vi "Stage_1_waveform_for_DAQ.vi"(11 "input cluster":T2) -> (2 "DAQ cluster":T1, 3 "Time cluster":cluster{"Total time":dbl, "Time per step":dbl})   [LabVIEW 2016]
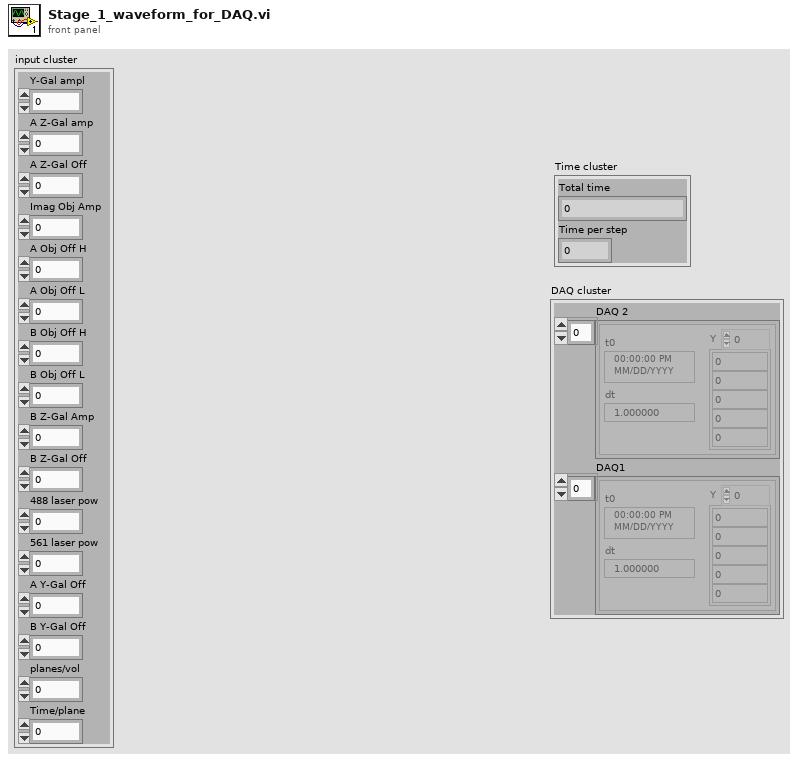
[diagram p1: front panel]
types:
  T1 = cluster{"DAQ1":waveform(dbl)[], "DAQ 2":waveform(dbl)[]}
  T2 = cluster{"Y-Gal ampl":dbl, "A Z-Gal amp":dbl, "A Z-Gal Off":dbl, "Imag Obj Amp":dbl, "A Obj Off H":dbl, "A Obj Off L":dbl, "B Obj Off H":dbl, "B Obj Off L":dbl, "B Z-Gal Amp":dbl, "B Z-Gal Off":dbl, "488 laser pow":dbl, "561 laser pow":dbl, "A Y-Gal Off":dbl, "B Y-Gal Off ":dbl, "planes/vol":dbl, "Time/plane":dbl}
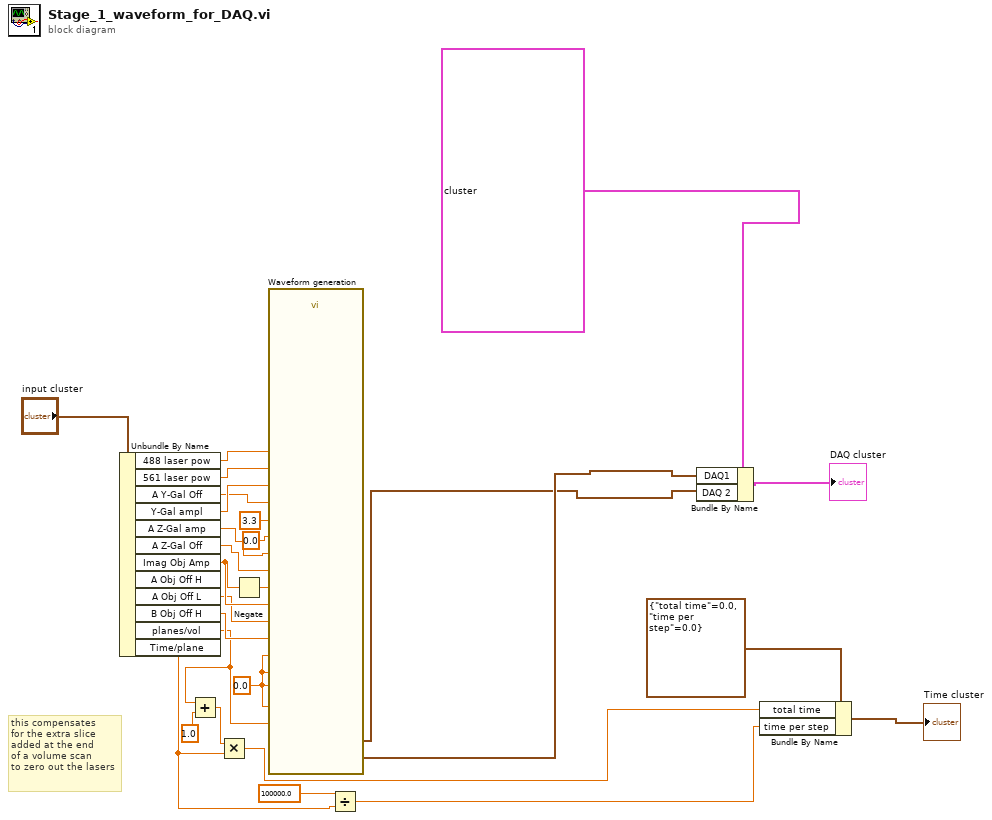
[diagram p0: block diagram]
diagram:
  w27 = 0.0 ("ARM2 Z-offset")
  # "this compensates\nfor the extra slice\nadded at the end\nof a volume scan\nto zero out the lasers"
  n1 = Unbundle By Name("input cluster") -> ("488 laser pow"=w14:dbl, "561 laser pow"=w15:dbl, "A Y-Gal Off"=w16:dbl, "Y-Gal ampl"=w22:dbl, "A Z-Gal amp"=w21:dbl, "A Z-Gal Off"=w20:dbl, "Imag Obj Amp"=w19:dbl, "A Obj Off L"=w18:dbl, "B Obj Off H"=w17:dbl, "planes/vol"=w12:dbl, "Time/plane"=w13:dbl)  [unwired: 1 out]
  n2 = Add(x=w12, y=1.0) -> (x+y=w11:dbl)
  n3 = Multiply(x=w11, y=w13) -> (x*y=w7:dbl)
  n4 = Negate(x=w19) -> (-x=w23:dbl)
  n5 = call "Waveform generation.vi"("Number of Steps"=w12, "488 LASER Intensity"=w14, "SPIMA Obj Ampl"=w23, "SPIMB Z- galvo amplitude"=w27, "SPIMA Z-Galvo Offset"=w20, "SPIMA Z-Galvo Amplitude"=w21, "SPIMA Camera trigger"=0.0 ("ARM2 Camera trigger"), "SPIMA Objective Offset"=w18, "SPIMB Objective Offset"=w17, "SPIMA Y-Galvo Offset"=w16, "SPIMB Camera Trigger"=3.3 ("ARM1 Camera Trigger"), "561 Laser Amplitude"=w15, "SPIMB Objective Amplitude"=w19, "SPIMA Y-Galvo Amplitude"=w22, "SPIMB Z-offset"=w27, "SPIMB Y Offset"=w27, "SPIMB Y Amplitude"=w27) -> ("DAQ 2"=w1:waveform(dbl)[], "DAQ1"=w2:waveform(dbl)[])  [unwired: 9 in]
  n6 = Divide(x=100000.0, y=w13) -> (x/y=w6:dbl)
  n7 = Bundle By Name(cluster=T1 {"DAQ1"=[{"t0"=timestamp(0 s since 1904-01-01), "dt"=1.0, "Y"=[0.0]}, {"t0"=timestamp(0 s since 1904-01-01), "dt"=1.0, "Y"=[0.0]}, {"t0"=timestamp(0 s since 1904-01-01), "dt"=1.0, "Y"=[0.0]}, {"t0"=timestamp(0 s since 1904-01-01), "dt"=1.0, "Y"=[0.0]}, {"t0"=timestamp(0 s since 1904-01-01), "dt"=1.0, "Y"=[0.0]}, {"t0"=timestamp(0 s since 1904-01-01), "dt"=1.0, "Y"=[0.0]}], "DAQ 2"=[{"t0"=timestamp(0 s since 1904-01-01), "dt"=1.0, "Y"=[0.0]}, {"t0"=timestamp(0 s since 1904-01-01), "dt"=1.0, "Y"=[0.0]}, {"t0"=timestamp(0 s since 1904-01-01), "dt"=1.0, "Y"=[0.0]}, {"t0"=timestamp(0 s since 1904-01-01), "dt"=1.0, "Y"=[0.0]}, {"t0"=timestamp(0 s since 1904-01-01), "dt"=1.0, "Y"=[0.0]}]}, "DAQ1"=w2, "DAQ 2"=w1) -> (→"DAQ cluster":T1)
  n8 = Bundle By Name(cluster=cluster{"total time":dbl, "time per step":dbl} {"total time"=0.0, "time per step"=0.0}, "total time"=w7, "time per step"=w6) -> (→"Time cluster":cluster{"total time":dbl, "time per step":dbl})
